vi "picoharp_write_lag_settings.vi"(8 "error in (no error)":errorcluster, 10 "lag_settings":T1 {"Lag Settings"."time_start" items=["1 ps"=1, "10 ps"=10, "100 ps"=100, "1 ns"=1000, "10 ns"=10000, "100 ns"=100000, "1 us"=1000000, "10 us"=10000000, "100 us"=100000000, "1 ms"=1000000000, "10 ms"=10000000000, "100 ms"=100000000000, "1 s"=1000000000000, "10 s"=10000000000000, "100 s"=100000000000000]; "Lag Settings"."time_end" items=["1 ps"=1, "10 ps"=10, "100 ps"=100, "1 ns"=1000, "10 ns"=10000, "100 ns"=100000, "1 us"=1000000, "10 us"=10000000, "100 us"=100000000, "1 ms"=1000000000, "10 ms"=10000000000, "100 ms"=100000000000, "1 s"=1000000000000, "10 s"=10000000000000, "100 s"=100000000000000]}, 11 "hydraharp in":refnum<class "picoharp.lvclass">) -> (0 "error out":errorcluster, 3 "hydraharp out":refnum<class "picoharp.lvclass">)   [LabVIEW 2015, in "picoharp.lvclass"]
uses:
  picoharp.lvclass
  Hydraharp/hydraharp_panel/hpanel_correlation_settings.ctl
  Hydraharp/hydraharp/hydraharp_correlation_lag_settings.ctl
  Hydraharp/hydraharp/hydraharp_time_decades.ctl
  picoharp.lvclass/picoharp.ctl
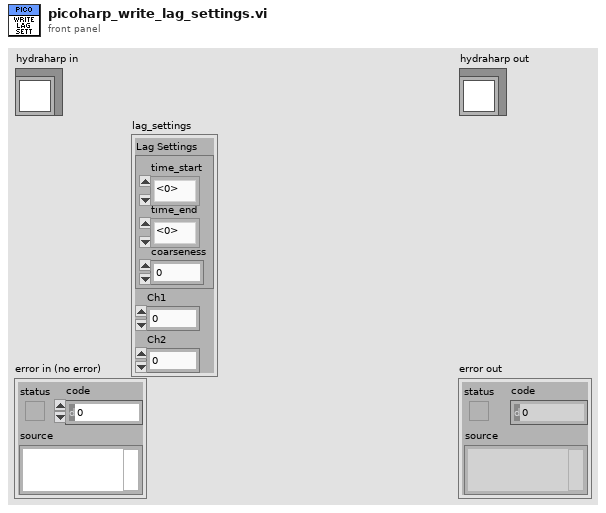
[diagram p1: front panel]
types:
  T1 = typedef "hpanel_correlation_settings.ctl" = cluster{"Lag Settings":T2, "Ch1":u8, "Ch2":u8}
  T2 = typedef "hydraharp_correlation_lag_settings.ctl" = cluster{"time_start":T3, "time_end":T3, "coarseness":i64}
  T3 = typedef "hydraharp_time_decades.ctl" = i64
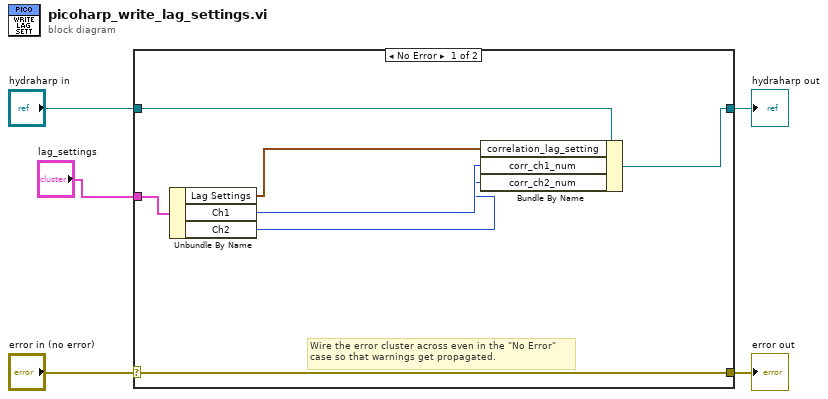
[diagram p0: block diagram]
diagram:
  n1 = case shown="No Error" "error in (no error)" {
    selector: "error in (no error)" -> [w12 w14]
    tunnel: [w12 w14] -> w4
    tunnel: [w6 w13] -> w2
    tunnel: "hydraharp in" -> [w11 w13]
    tunnel: "lag_settings" -> [w10 _]
    frame No Error {
      # "Wire the error cluster across even in the \"No Error\"\ncase so that warnings get propagated."
      n2 = Unbundle By Name(w10) -> ("Lag Settings"=w9:T2, "Ch1"=w8:u8, "Ch2"=w7:u8)
      n3 = Bundle By Name(cluster=w11, "correlation_lag_setting"=w9, "corr_ch1_num"=w8, "corr_ch2_num"=w7) -> (w6:refnum<class "picoharp.lvclass">)
    }
    frame Error {
    }
  }
  "error out" <- w4
  "hydraharp out" <- w2
